vi "DAQ@Calculate__Parameter.vi"(1 "ParamterIn":string) -> (0 "ParamterOut":string)   [LabVIEW 2020]
panel:
  out "WaveFormNameList":string[](array[string])
  in  "WaveFormA":string(combo)
  in  "Confirm":bool
  # "Move         $WaveFormA=$WaveFormB\nAppend       $WaveFormA<=$WaveFormB\nAdd           $WaveFormA=$WaveFormB + $WaveFormC\nSub           $WaveFormA=$WaveFormB - $WaveFormC\nMul           $WaveFormA=$WaveFormB * $WaveFormC\nDiv            $WaveFormA=$WaveFormB / $WaveFormC\nConv         $WaveFormA=$WaveFormB @ $WaveFormC\nSection       $WaveFormA=$WaveFormB%[$TIME0~$TIME1]\nDiff            $WaveFormA $= $WaveFormB\nSerialize      $WaveFormA <<= $WaveFormB"
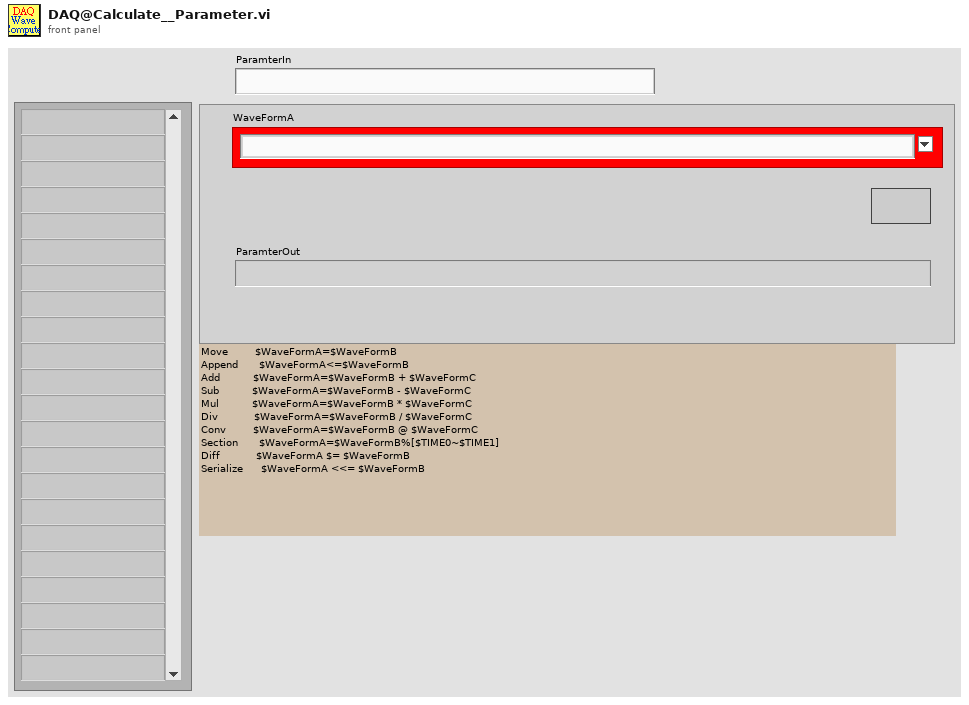
[diagram p1: front panel]
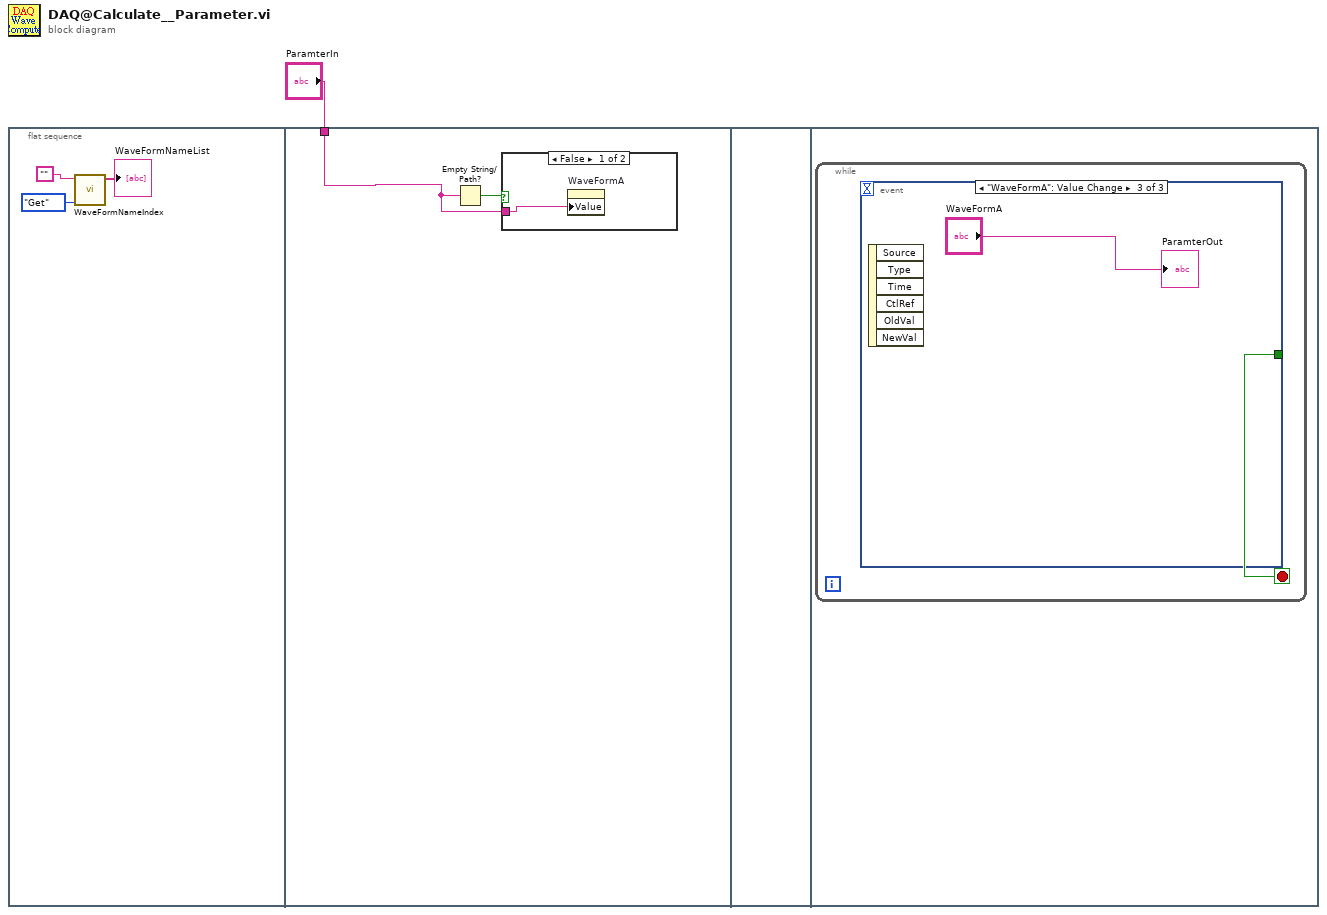
[diagram p0: block diagram]
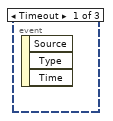
[diagram p3: hidden frame]
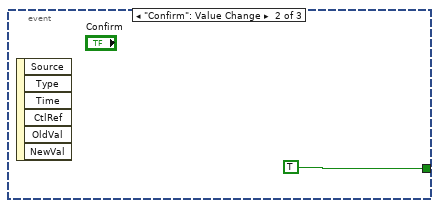
[diagram p4: hidden frame]
diagram:
  n1 = flat-sequence {
    tunnel: "ParamterIn" -> [w5]
    frame #0 {
      n2 = call "WaveFormNameIndex.vi"("OP"=enum16{"Get", "Update", "Init", "GetSPS"}."Get", "WaveFormName"="") -> ("WaveFormNameList"=→"WaveFormNameList":string[])  [unwired: 6 in, 3 out]
    }
    frame #1 {
      n3 = Empty String/Path?(string/path=w5) -> (empty?=w6:bool)
      n4 = case shown="False" w6 {
        tunnel: w5 -> [w7 _]
        frame False {
          n5 = property on="WaveFormA" class="CmbBox"("Value"=w7) -> ()  [unwired: 2 in, 2 out]
        }
        frame True {
        }
      }
    }
    frame #2 {
    }
    frame #3 {
      n6 = while {
        stop <- w8 stop-if-true
        n7 = event shown="[2] \"WaveFormA\": Value Change" {
          selector: _ -> [_ _ _]
          dyn-events: _ -> [_ _ _]
          timeout: _ -> [_ _ _]
          tunnel: [_ TRUE _] -> w8
          event Timeout {
            n8 = event-data() -> ()  [unwired: 1 in, 3 out]
          }
          event "Confirm": Value Change {
            n9 = event-data() -> ()  [unwired: 1 in, 6 out]
          }
          event "WaveFormA": Value Change {
            n10 = event-data() -> ()  [unwired: 1 in, 6 out]
            "ParamterOut" <- "WaveFormA"
          }
        }
      }
    }
  }
